vi "PIO.Read (I64).vi"(8 "error in (no error)":errorcluster, 10 "offset":u32 format="%.0x", 11 "GE 5565PIORC in":refnum<class "GE 5565PIORC Old.lvclass">) -> (0 "error out":errorcluster, 2 "value":i64, 3 "GE 5565PIORC out":refnum<class "GE 5565PIORC Old.lvclass">)   [LabVIEW 2016, in "GE 5565PIORC Old.lvclass"]
uses:
  GE 5565PIORC Old.lvclass
  GE 5565PIORC Old.lvclass/GE 5565PIORC Old.ctl
  SubVIs/Change Endianness (U64).vi
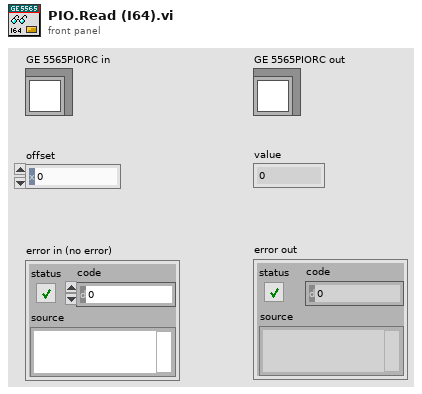
[diagram p1: front panel]
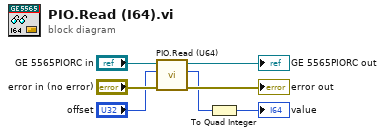
[diagram p0: block diagram]
diagram:
  n1 = call "PIO.Read (U64).vi"("error in (no error)"="error in (no error)", "offset"="offset", "GE 5565PIORC in"="GE 5565PIORC in") -> ("error out"=→"error out":errorcluster, "value"=w1:u64, "GE 5565PIORC out"=→"GE 5565PIORC out":refnum<class "GE 5565PIORC Old.lvclass">)  [unwired: 6 in]
  n2 = To Quad Integer(1:w1) -> (0:→"value":i64)
